vi "SoundOutput.vi"() -> ()   [LabVIEW 2014]
uses:
  <vilib>/sound2/lvsound2.llb/Sound Data Format.ctl
  <vilib>/sound2/lvsound2.llb/Sampling Mode.ctl
  <vilib>/sound2/lvsound2.llb/Sound Output Write (DBL Single).vi
  <vilib>/measure/NI_MABase.lvlib
panel:
  in  "duty cycle (%)":dbl=50.0 format="%0.2f"
  out "Waveform Graph":waveform(dbl)(graph)
  in  "amplitude":dbl=1.0 format="%0.2p"
  in  "frequency":dbl=10.0 format="%0.2p"
  in  "stop":bool
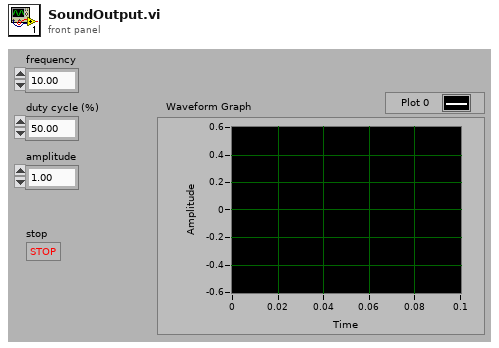
[diagram p1: front panel]
types:
  T1 = typedef "Sampling Mode.ctl" = i32
  T2 = typedef "Sound Data Format.ctl" = cluster{"sample rate (S/s)":dbl, "number of channels":i32, "bits per sample":i32}
  T3 = typedef "Sound Output Task ID.ctl" = u32
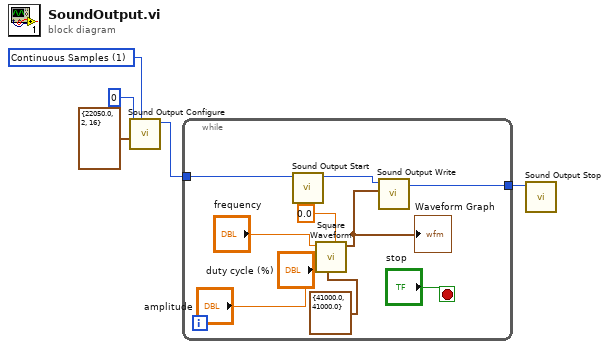
[diagram p0: block diagram]
diagram:
  w3 = T1 1 items=["Finite Samples", "Continuous Samples"] ("sample mode")
  n1 = call <vilib>:"Sound Output Configure.vi"("sample mode"=w3, "sound format"=T2 {"sample rate (S/s)"=22050.0, "number of channels"=2, "bits per sample"=16}, "device ID"=u32 0) -> ("task ID"=w2:T3)  [unwired: 7 in, 1 out]
  n2 = while {
    tunnel: w2 -> [w14]
    tunnel: [w12] -> w1
    stop <- "stop" stop-if-true
    n3 = call <vilib>:"Sound Output Start.vi"("task ID"=w14) -> ("task ID out"=w13:T3)  [unwired: 9 in, 1 out]
    n4 = call <vilib>:"Square Waveform.vi"("duty cycle (%)"="duty cycle (%)", "offset"=0.0, "sampling info"=cluster{"Fs":dbl, "#s":dbl} {"Fs"=41000.0, "#s"=41000.0}, "amplitude"="amplitude", "frequency"="frequency") -> ("signal out"=w7:waveform(dbl))  [unwired: 5 in, 1 out]
    "Waveform Graph" <- w7
    n5 = call-poly <vilib>:"Sound Output Write.vi"("data"=w7, "task ID"=w13) -> ("task ID out"=w12:T3)  [unwired: 8 in, 1 out]
  }
  n6 = call <vilib>:"Sound Output Stop.vi"("task ID"=w1) -> ()  [unwired: 9 in, 2 out]
